vi "Test Create Multiple Reports.vi"(8 "error in (no error)":errorcluster, 11 "XML Report Test in":refnum<class "XML Report Test.lvclass">) -> (0 "error out":errorcluster, 3 "XML Report Test out":refnum<class "XML Report Test.lvclass">)   [LabVIEW 2020, in "XML Report Test.lvclass"]
uses:
  XML Report Test.lvclass
  C:/Program Files (x86)/National Instruments/LabVIEW 2020/vi.lib/Astemes/LUnit/Test Case.lvclass
  source/Plugins/XML Report/XML Report.lvclass
  XML Report Test.lvclass/XML Report Test.ctl
  <vilib>/Astemes/LUnit/Test Case.lvclass/Test Case.ctl
  <vilib>/Astemes/LUnit/Palette/Pass.vi
  <vilib>/Astemes/LUnit/Palette/Fail.vi
  <vilib>/Astemes/LUnit/Set Assertion Type.vi
  <vilib>/Astemes/LUnit/Add test result.vi
  <vilib>/Astemes/LUnit/LUnit Record Assertion Result.vi
  <vilib>/Astemes/LUnit/LUnit Aggregate Assertion Results.vi
  <vilib>/Astemes/LUnit/Method Result/LUnit Merge Status.vi
  <vilib>/Astemes/LUnit/LUnit Concatenate result strings.vi
  <vilib>/Astemes/LUnit/Test Case.lvclass
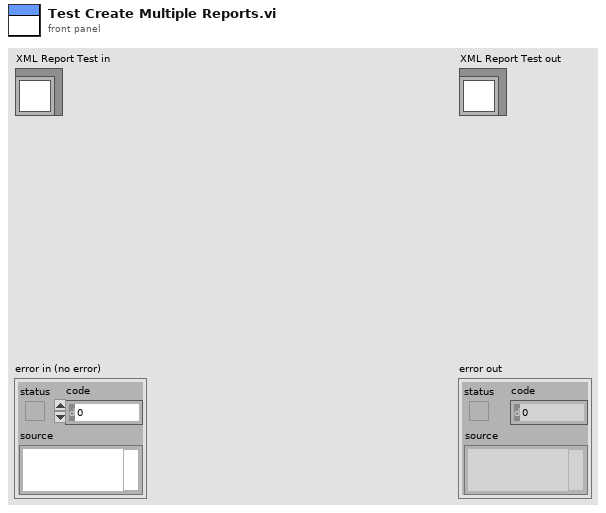
[diagram p1: front panel]
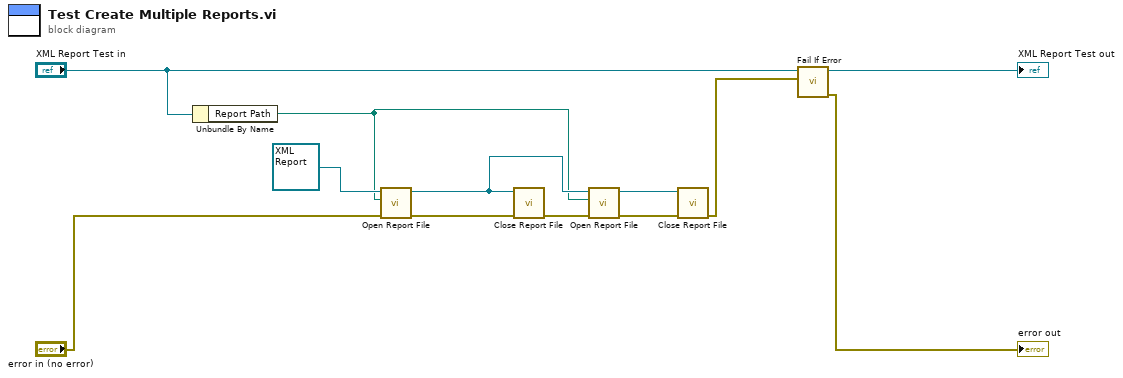
[diagram p0: block diagram]
diagram:
  n1 = Unbundle By Name("XML Report Test in") -> ("Report Path"=w1:path)
  n2 = call-dynamic "Open Report File.vi"("error in (no error)"="error in (no error)", "Report Path"=w1, "XML Report In"=refnum<class "XML Report.lvclass"> refnum) -> ("error out"=w12:errorcluster, "XML Report Out"=w3:refnum<class "XML Report.lvclass">)  [unwired: 7 in]
  n3 = call-dynamic "Close Report File.vi"("error in (no error)"=w12, "XML Report In"=w3) -> ("error out"=w4:errorcluster)  [unwired: 8 in, 1 out]
  n4 = call-dynamic "Open Report File.vi"("error in (no error)"=w4, "Report Path"=w1, "XML Report In"=w3) -> ("error out"=w5:errorcluster, "XML Report Out"=w6:refnum<class "XML Report.lvclass">)  [unwired: 7 in]
  n5 = call-dynamic "Close Report File.vi"("error in (no error)"=w5, "XML Report In"=w6) -> ("error out"=w2:errorcluster)  [unwired: 8 in, 1 out]
  n6 = call <vilib>:"Fail If Error.vi"("Assert error"=w2, "LUnit Test Case In"="XML Report Test in") -> ("error out"=→"error out":errorcluster, "LUnit Test Case Out"=→"XML Report Test out":refnum<class "XML Report Test.lvclass">)  [unwired: 8 in]
